vi "Convert Fm to 2D array.vi"(0 "Data in":dbl[][](array[numeric]), 1 "Data Cluster":T1) -> (5 "Scalar data":dbl, 6 "Data out":dbl[][](array[numeric]))   [LabVIEW 2019]
uses:
  controls/UI Data.ctl
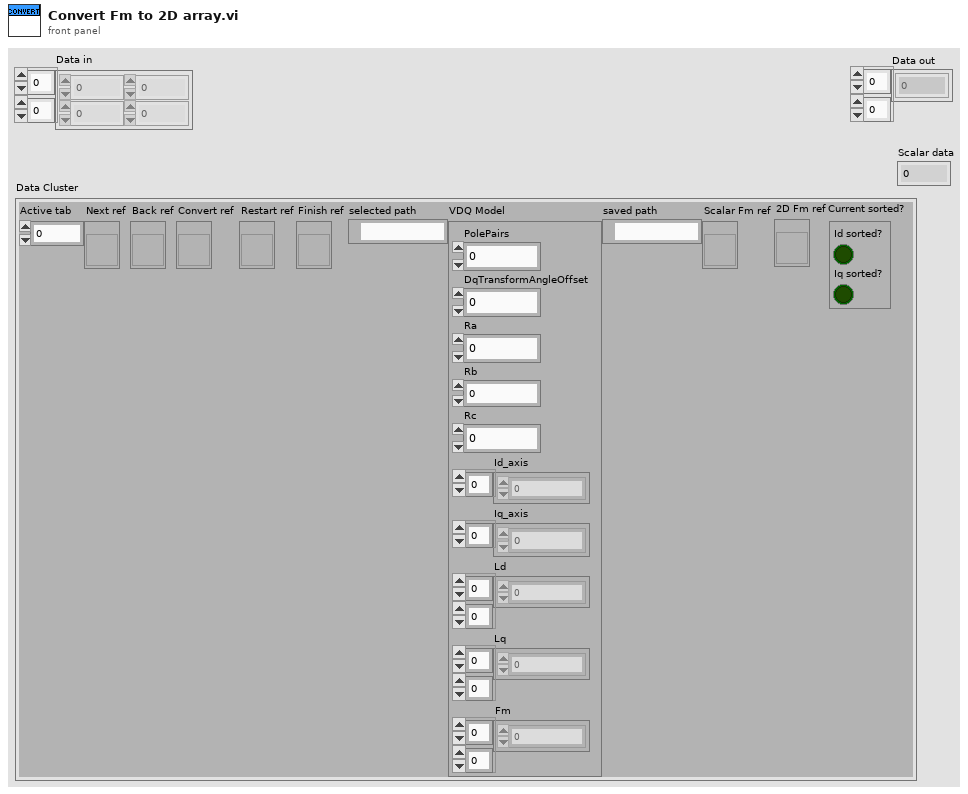
[diagram p1: front panel]
types:
  T1 = typedef "UI Data.ctl" = cluster{"Active tab":u32, "Next ref":refnum<vi>, "Back ref":refnum<vi>, "Convert ref":refnum<vi>, "Restart ref":refnum<vi>, "Finish ref":refnum<vi>, "selected path":path, "VDQ Model":cluster{"PolePairs":dbl, "DqTransformAngleOffset":dbl, "Ra":dbl, "Rb":dbl, "Rc":dbl, "Id_axis":dbl[], "Iq_axis":dbl[], "Ld":dbl[][], "Lq":dbl[][], "Fm":dbl[][]}, "saved path":path, "Scalar Fm ref":refnum<vi>, "2D Fm ref":refnum<vi>, "Current sorted?":cluster{"Id sorted?":bool, "Iq sorted?":bool}}
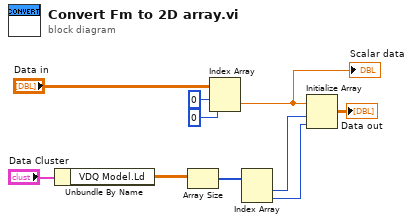
[diagram p0: block diagram]
diagram:
  n1 = Unbundle By Name("Data Cluster") -> ("VDQ Model.Ld"=w1:dbl[][])
  n2 = Array Size(array=w1) -> (size(s)=w6:i32[])
  n3 = Index Array(array="Data in", index (row)=0, index (col)=0 ("disabled index (col)")) -> (element=w7:dbl)
  "Scalar data" <- w7
  n4 = Index Array(array=w6) -> (element #1=w5:i32, element #2=w4:i32)  [unwired: 2 in]
  n5 = Initialize Array(w7, w5, w4) -> (→"Data out":dbl[][])
